vi "Main.vi"(11 "Error in":errorcluster) -> (15 "Error out":errorcluster)   [LabVIEW 2020, in "Simple calculator.lvlib"]
doc: "This System is an advanced calculator which is used to store and retrive data which we have already made."
uses:
  Simple calculator.lvlib
  Typedefs/Queue operations.ctl
  Typedefs/Data cluster.ctl
  Arithmetic Operations/Add/Add.lvclass
  Arithmetic Operations/Subtract/Subtract.lvclass
  Arithmetic Operations/Multiply/Multiply.lvclass
  Arithmetic Operations/Divide/Divide.lvclass
  Typedefs/User event operations.ctl
panel:
  in  "Delete":bool
  in  "Load":bool
  in  "Save":bool
  in  "Arithmetic operation":string(combo)
  in  "Add":bool
  in  "Operations added":string(tree)
  # "ADVANCED CALCULATOR"
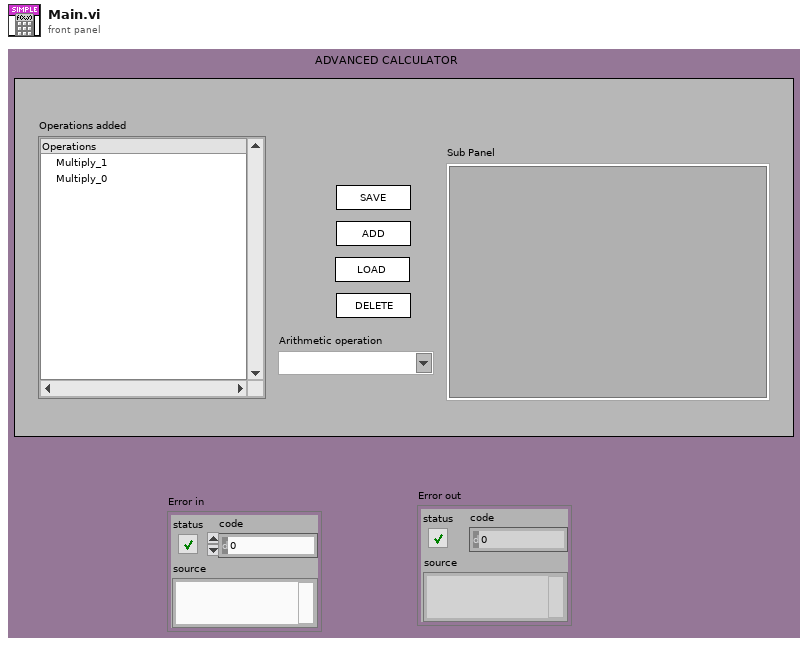
[diagram p1: front panel]
types:
  T1 = typedef "Simple calculator.lvlib/User event operations.ctl" = enum16{"Create", "Get Ref", "Generate ", "Destroy"}
  T2 = typedef "Simple calculator.lvlib/Data cluster.ctl" = cluster{"Load":bool, "Save":bool, "Add":bool, "Arithmetic operation":string, "Add Count":dbl, "Subtract Count":dbl, "Multiply Count":dbl, "Divide Count":dbl, "Delete Tag":string, "Add Object":refnum<class "Add.lvclass">[], "Sub Object":refnum<class "Subtract.lvclass">[], "Multiply Object":refnum<class "Multiply.lvclass">[], "Divide Object":refnum<class "Divide.lvclass">[], "Previous tag":i32, "Strict VI Ref":refnum<vi>, "Active Tag":i32, "Sub VI Refnum":refnum<vi>, "Multip VI Refnum":refnum<vi>, "Divide vi refnum":refnum<vi>}
  T3 = typedef "Simple calculator.lvlib/Queue operations.ctl" = enum16{"Create", "Enqueue", "Enstack", "Dequeue", "Flush", "Release"}
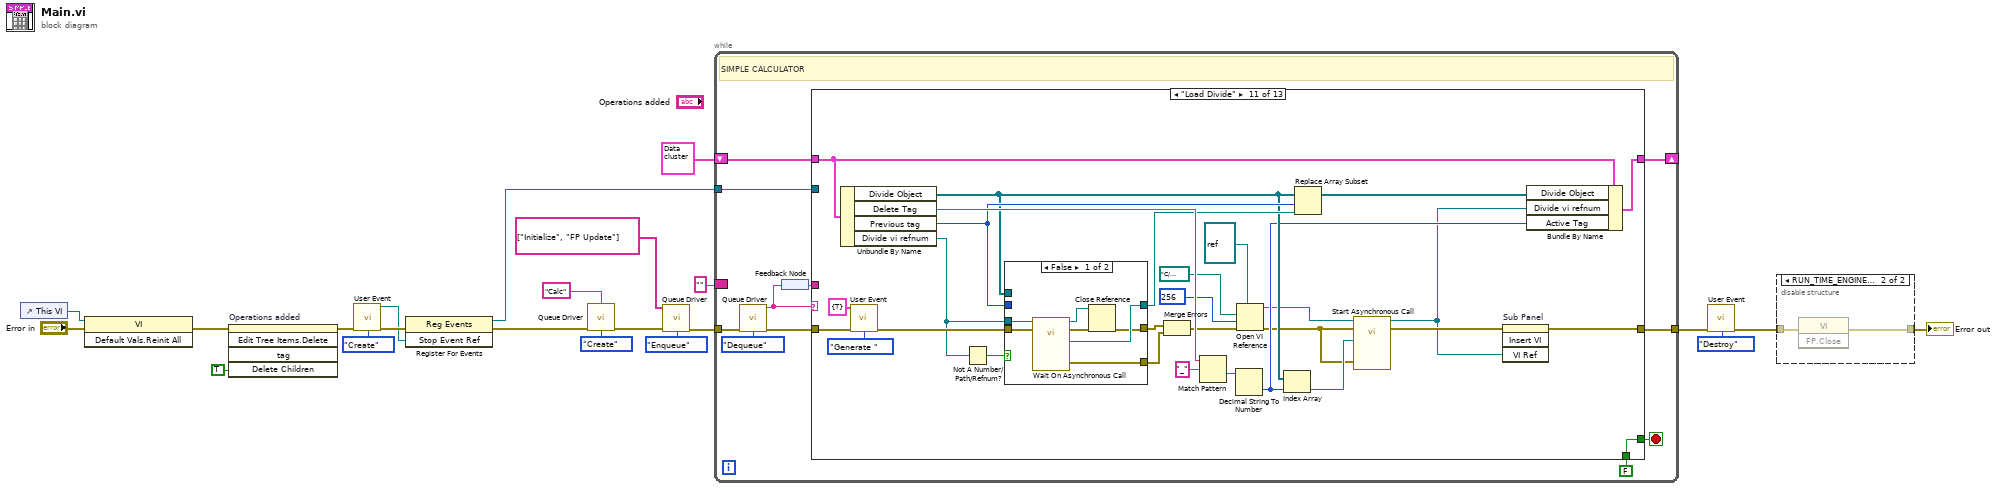
[diagram p0: block diagram]
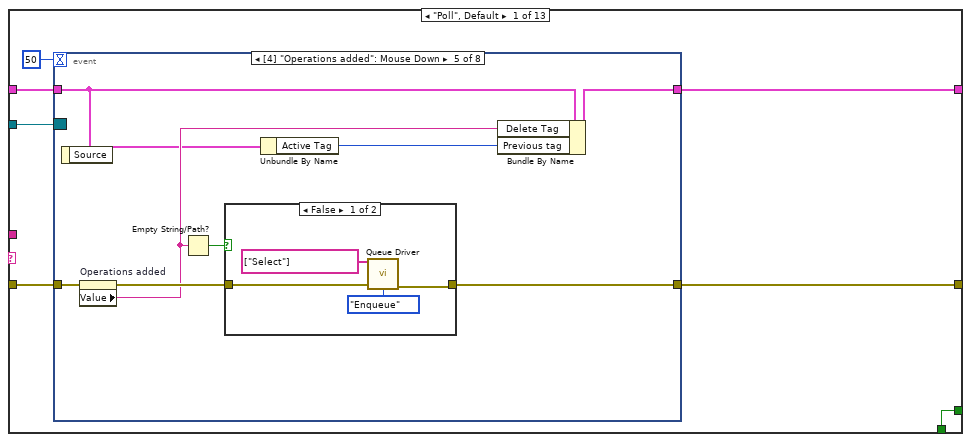
[diagram p3: hidden frame]
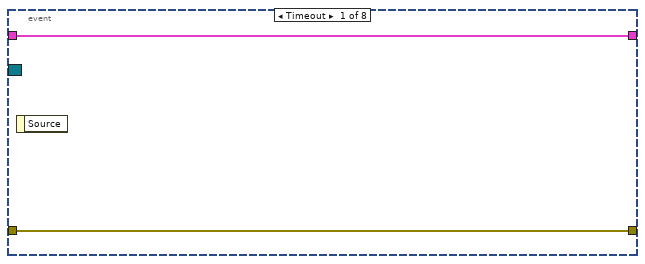
[diagram p4: hidden frame]
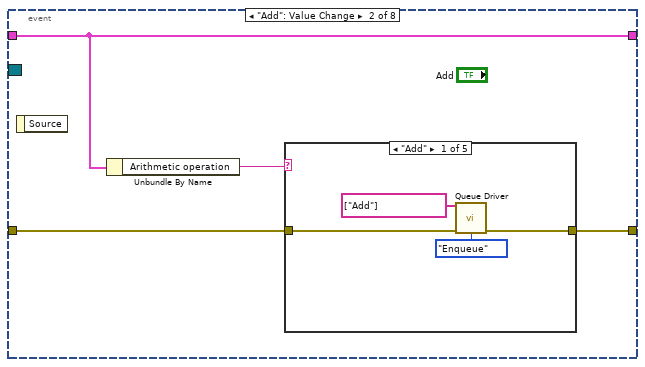
[diagram p5: hidden frame]
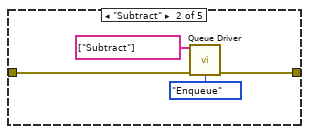
[diagram p6: hidden frame]
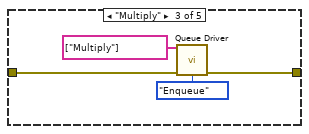
[diagram p7: hidden frame]
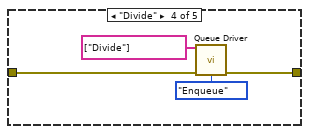
[diagram p8: hidden frame]
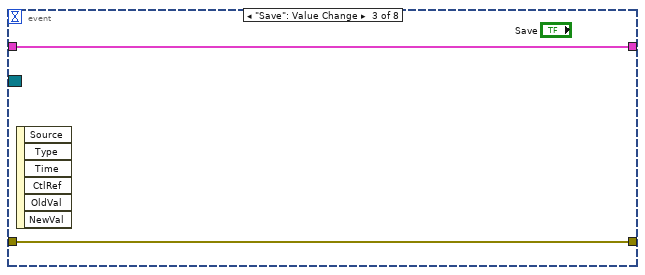
[diagram p10: hidden frame]
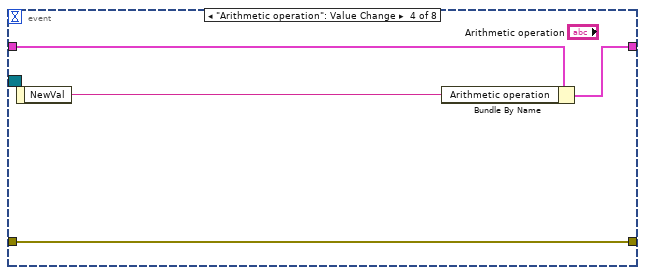
[diagram p11: hidden frame]
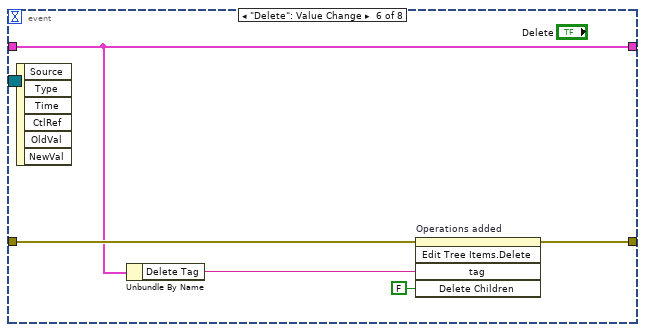
[diagram p13: hidden frame]
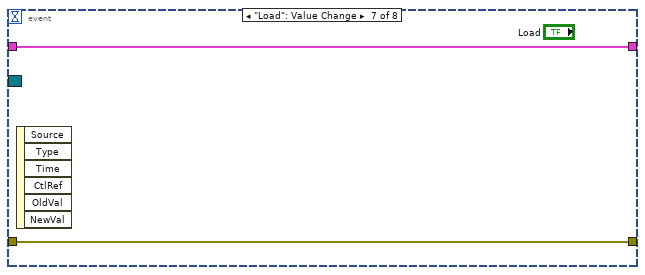
[diagram p14: hidden frame]
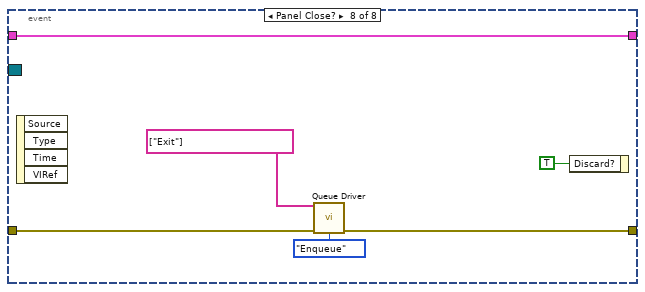
[diagram p15: hidden frame]
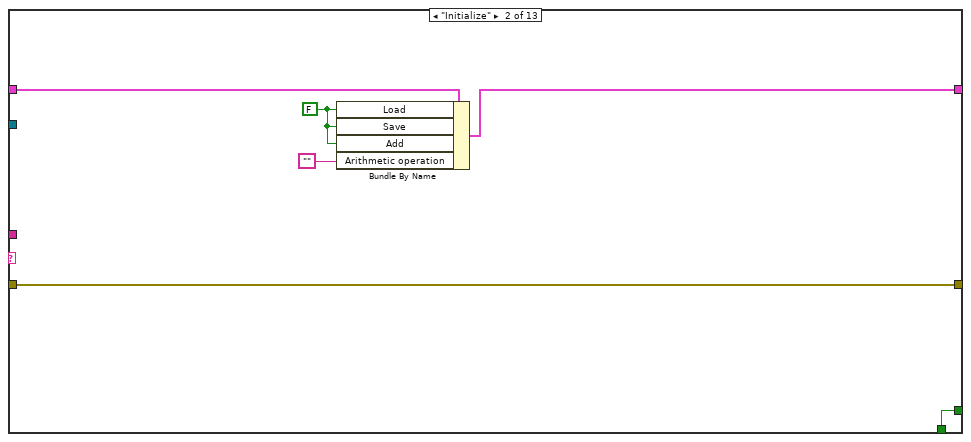
[diagram p16: hidden frame]
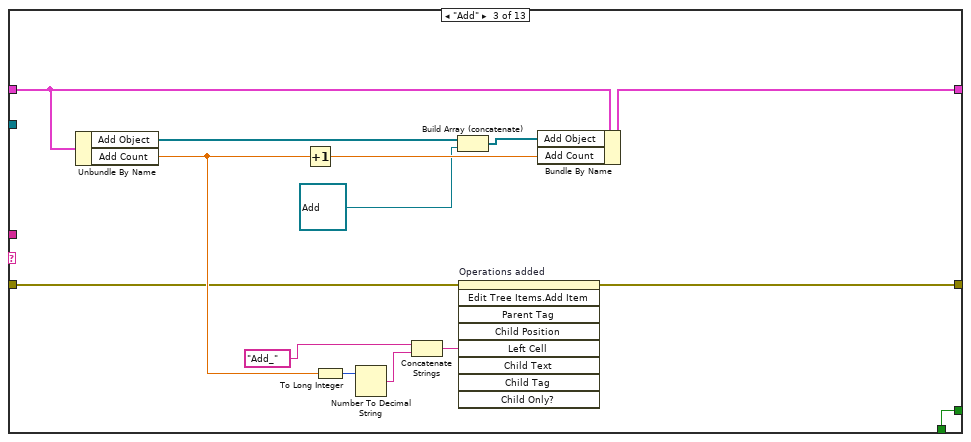
[diagram p17: hidden frame]
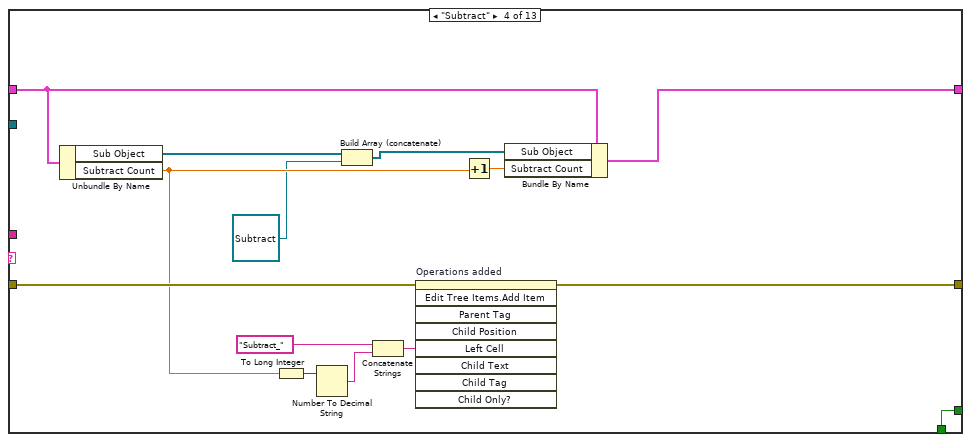
[diagram p18: hidden frame]
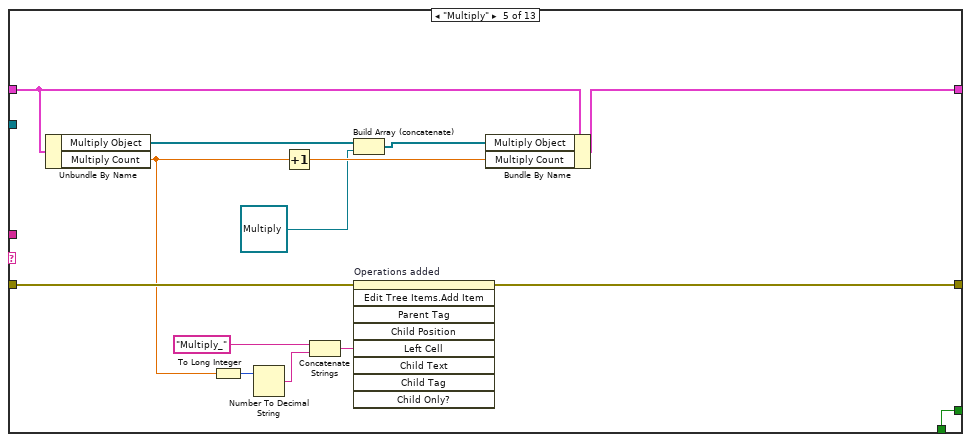
[diagram p19: hidden frame]
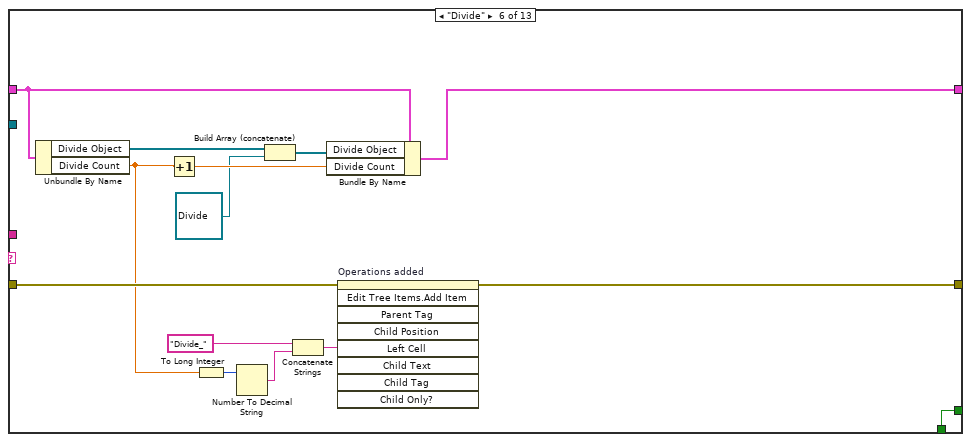
[diagram p20: hidden frame]
diagram:
  n1 = control-ref of="This VI"() -> (w21:refnum<vi>)
  n2 = invoke class="VI" method="Default Vals.Reinit All"(reference=w21, error in="Error in") -> (error out=w2:errorcluster)  [unwired: 1 in, 2 out]
  n3 = invoke on="Operations added" class="Tree (strict)" method="Edit Tree Items.Delete"(error in=w2, "Delete Children"=TRUE ("Delete Children?")) -> (error out=w1:errorcluster)  [unwired: 3 in, 4 out]
  n4 = call "User Event.vi"("Error in"=w1, "Operation"=User_event_operations."Create") -> ("Stop Event Ref"=w8:refnum<user-event>, "Error out"=w10:errorcluster)  [unwired: 12 in]
  n5 = register-events(error in=w10, w8) -> (reference out=w7:refnum<event-registration>, error out=w9:errorcluster)  [unwired: 1 in]
  n6 = call "Queue Driver.vi"("Name"="Calc", "Error in"=w9, "Operations"=Queue_operations."Create") -> ("Error out"=w17:errorcluster)  [unwired: 11 in, 1 out]
  n7 = call "Queue Driver.vi"("Enqueue states"=string[] ["Initialize", "FP Update"], "Error in"=w17, "Operations"=Queue_operations."Enqueue") -> ("Error out"=w15:errorcluster)  [unwired: 11 in, 1 out]
  n8 = while {
    tunnel: w15 -> [w32]
    border: "" ("Dequeued element") -> [_]
    tunnel: [w28] -> w5
    shift-right: [w25] -> _
    shift-left: T2 {"Load"=FALSE, "Save"=FALSE, "Add"=FALSE, "Arithmetic operation"="", "Add Count"=0.0, "Subtract Count"=0.0, "Multiply Count"=0.0, "Divide Count"=0.0, "Delete Tag"="", "Add Object"=[], "Sub Object"=[], "Multiply Object"=[], "Divide Object"=[], "Previous tag"=0, "Strict VI Ref"=refnum, "Active Tag"=0, "Sub VI Refnum"=refnum, "Multip VI Refnum"=refnum, "Divide vi refnum"=refnum} -> [w24]
    tunnel: w7 -> [w23]
    stop <- w27 stop-if-true
    # "SIMPLE CALCULATOR"
    n9 = call "Queue Driver.vi"("Error in"=w32, "Operations"=Queue_operations."Dequeue") -> ("Dequeued element"=w31:string, "Error out"=w29:errorcluster)  [unwired: 12 in]
    n10 = feedback-in #1(w31) -> ()
    n11 = feedback #1() -> (w30:string)
    n12 = case shown="\"Load Divide\"" w31 {
      tunnel: w30 -> [_ _ _ _ _ _ _ _ _ _ _ w346 _]
      tunnel: w29 -> [w40 w101 w103 w125 w142 w156 w159 w191 w223 w287 w327 w347 w363]
      tunnel: [w39 w101 w111 w124 w141 w155 w158 w187 w249 w262 w303 w343 w367] -> w28
      tunnel: [w38 w100 w115 w129 w143 w157 w164 w210 w250 w290 w330 w355 TRUE] -> w27
      tunnel: FALSE -> [w38 w100 w115 w129 w143 w157 w164 w210 w250 w290 w330 w355 _]
      tunnel: [w35 w98 w108 w119 w135 w149 w163 w201 w240 w274 w314 w342 w365] -> w25
      tunnel: w24 -> [w36 w99 w110 w120 w136 w150 w163 w202 w241 w275 w315 w342 w365]
      tunnel: w23 -> [w34 _ _ _ _ _ _ _ _ _ _ _ _]
      frame "Poll", Default {
        n13 = event shown="[4] \"Operations added\": Mouse Down" {
          selector: w34 -> [_ _ _ _ _ _ _ _]
          dyn-events: _ -> [_ _ _ _ _ _ _ _]
          timeout: 50 -> [_ _ _ _ _ _ _ _]
          tunnel: w40 -> [w42 w44 w65 w69 w77 w87 w89 w93]
          tunnel: [w42 w43 w65 w69 w70 w86 w89 w92] -> w39
          tunnel: w36 -> [w41 w46 w64 w68 w72 w84 w88 w90]
          tunnel: [w41 w46 w64 w66 w76 w84 w88 w90] -> w35
          event Timeout {
            n14 = event-data() -> ()  [unwired: 1 in, 1 out]
          }
          event "Add": Value Change {
            n15 = event-data() -> ()  [unwired: 1 in, 1 out]
            n16 = Unbundle By Name(w46) -> ("Arithmetic operation"=w45:string)
            n17 = case shown="\"Add\"" w45 {
              tunnel: w44 -> [w49 w52 w56 w60 w63]
              tunnel: [w47 w51 w55 w59 w63] -> w43
              frame "Add" {
                n18 = call "Queue Driver.vi"("Enqueue states"=string[] ["Add"], "Error in"=w49, "Operations"=Queue_operations."Enqueue") -> ("Error out"=w47:errorcluster)  [unwired: 11 in, 1 out]
              }
              frame "Subtract" {
                n19 = call "Queue Driver.vi"("Enqueue states"=string[] ["Subtract"], "Error in"=w52, "Operations"=Queue_operations."Enqueue") -> ("Error out"=w51:errorcluster)  [unwired: 11 in, 1 out]
              }
              frame "Multiply" {
                n20 = call "Queue Driver.vi"("Enqueue states"=string[] ["Multiply"], "Error in"=w56, "Operations"=Queue_operations."Enqueue") -> ("Error out"=w55:errorcluster)  [unwired: 11 in, 1 out]
              }
              frame "Divide" {
                n21 = call "Queue Driver.vi"("Enqueue states"=string[] ["Divide"], "Error in"=w60, "Operations"=Queue_operations."Enqueue") -> ("Error out"=w59:errorcluster)  [unwired: 11 in, 1 out]
              }
              frame "", Default {
              }
            }
          }
          event "Save": Value Change {
            n22 = event-data() -> ()  [unwired: 1 in, 6 out]
          }
          event "Arithmetic operation": Value Change {
            n23 = event-data() -> ("NewVal"=w67:string)  [unwired: 1 in]
            n24 = Bundle By Name(cluster=w68, "Arithmetic operation"=w67) -> (w66:T2)
          }
          event "Operations added": Mouse Down {
            n25 = event-data() -> ()  [unwired: 1 in, 1 out]
            n26 = property on="Operations added" class="Tree (strict)"(error in=w77) -> (error out=w74:errorcluster, "Value"=w73:string)  [unwired: 1 in, 1 out]
            n27 = Empty String/Path?(string/path=w73) -> (empty?=w75:bool)
            n28 = case shown="False" w75 {
              tunnel: [w79 w82] -> w70
              tunnel: w74 -> [w80 w82]
              frame False {
                n29 = call "Queue Driver.vi"("Enqueue states"=string[] ["Select"], "Error in"=w80, "Operations"=Queue_operations."Enqueue") -> ("Error out"=w79:errorcluster)  [unwired: 11 in, 1 out]
              }
              frame True {
              }
            }
            n30 = Unbundle By Name(w72) -> ("Active Tag"=w71:i32)
            n31 = Bundle By Name(cluster=w72, "Delete Tag"=w73, "Previous tag"=w71) -> (w76:T2)
          }
          event "Delete": Value Change {
            n32 = event-data() -> ()  [unwired: 1 in, 6 out]
            n33 = Unbundle By Name(w84) -> ("Delete Tag"=w83:string)
            n34 = invoke on="Operations added" class="Tree (strict)" method="Edit Tree Items.Delete"(error in=w87, "tag"=w83, "Delete Children"=FALSE ("Delete Children?")) -> (error out=w86:errorcluster)  [unwired: 2 in, 4 out]
          }
          event "Load": Value Change {
            n35 = event-data() -> ()  [unwired: 1 in, 6 out]
          }
          event Panel Close? {
            n36 = event-data() -> ()  [unwired: 1 in, 4 out]
            n37 = call "Queue Driver.vi"("Enqueue states"=string[] ["Exit"], "Error in"=w93, "Operations"=Queue_operations."Enqueue") -> ("Error out"=w92:errorcluster)  [unwired: 11 in, 1 out]
            n38 = event-data("Discard?"=TRUE) -> ()  [unwired: 1 in, 1 out]
          }
        }
      }
      frame "Initialize" {
        w97 = FALSE ("Load")
        n39 = Bundle By Name(cluster=w99, "Load"=w97, "Save"=w97, "Add"=w97, "Arithmetic operation"="") -> (w98:T2)
      }
      frame "Add" {
        n40 = Unbundle By Name(w110) -> ("Add Object"=w105:refnum<class "Add.lvclass">[], "Add Count"=w107:dbl)
        n41 = Increment(x=w107) -> (x+1=w109:dbl)
        n42 = To Long Integer(number=w107) -> (32bit integer=w114:i32)
        n43 = Number To Decimal String(number=w114) -> (decimal integer string=w113:string)  [unwired: 1 in]
        n44 = Concatenate Strings("Add_" ("Arithmetic operation"), w113) -> (w112:string)
        n45 = Build Array (concatenate)(w105, refnum<class "Add.lvclass"> refnum ("Add.lvclass")) -> (w104:refnum<class "Add.lvclass">[])
        n46 = invoke on="Operations added" class="Tree (strict)" method="Edit Tree Items.Add Item"(error in=w103, "Left Cell"=w112) -> (error out=w111:errorcluster)  [unwired: 7 in, 8 out]
        n47 = Bundle By Name(cluster=w110, "Add Object"=w104, "Add Count"=w109) -> (w108:T2)
      }
      frame "Subtract" {
        n48 = Unbundle By Name(w120) -> ("Sub Object"=w118:refnum<class "Subtract.lvclass">[], "Subtract Count"=w122:dbl)
        n49 = To Long Integer(number=w122) -> (32bit integer=w128:i32)
        n50 = Number To Decimal String(number=w128) -> (decimal integer string=w126:string)  [unwired: 1 in]
        n51 = Build Array (concatenate)(w118, refnum<class "Subtract.lvclass"> refnum ("Subtract.lvclass")) -> (w116:refnum<class "Subtract.lvclass">[])
        n52 = Concatenate Strings("Subtract_" ("string"), w126) -> (w123:string)
        n53 = invoke on="Operations added" class="Tree (strict)" method="Edit Tree Items.Add Item"(error in=w125, "Left Cell"=w123) -> (error out=w124:errorcluster)  [unwired: 7 in, 8 out]
        n54 = Increment(x=w122) -> (x+1=w121:dbl)
        n55 = Bundle By Name(cluster=w120, "Sub Object"=w116, "Subtract Count"=w121) -> (w119:T2)
      }
      frame "Multiply" {
        n56 = Unbundle By Name(w136) -> ("Multiply Object"=w132:refnum<class "Multiply.lvclass">[], "Multiply Count"=w133:dbl)
        n57 = To Long Integer(number=w133) -> (32bit integer=w140:i32)
        n58 = Number To Decimal String(number=w140) -> (decimal integer string=w138:string)  [unwired: 1 in]
        n59 = Increment(x=w133) -> (x+1=w134:dbl)
        n60 = Concatenate Strings("Multiply_" ("string"), w138) -> (w137:string)
        n61 = Build Array (concatenate)(w132, refnum<class "Multiply.lvclass"> refnum ("Multiply.lvclass")) -> (w130:refnum<class "Multiply.lvclass">[])
        n62 = invoke on="Operations added" class="Tree (strict)" method="Edit Tree Items.Add Item"(error in=w142, "Left Cell"=w137) -> (error out=w141:errorcluster)  [unwired: 7 in, 8 out]
        n63 = Bundle By Name(cluster=w136, "Multiply Object"=w130, "Multiply Count"=w134) -> (w135:T2)
      }
      frame "Divide" {
        n64 = Unbundle By Name(w150) -> ("Divide Object"=w146:refnum<class "Divide.lvclass">[], "Divide Count"=w147:dbl)
        n65 = Increment(x=w147) -> (x+1=w148:dbl)
        n66 = To Long Integer(number=w147) -> (32bit integer=w154:i32)
        n67 = Number To Decimal String(number=w154) -> (decimal integer string=w152:string)  [unwired: 1 in]
        n68 = Build Array (concatenate)(w146, refnum<class "Divide.lvclass"> refnum ("Divide.lvclass")) -> (w144:refnum<class "Divide.lvclass">[])
        n69 = Concatenate Strings("Divide_" ("string"), w152) -> (w151:string)
        n70 = Bundle By Name(cluster=w150, "Divide Object"=w144, "Divide Count"=w148) -> (w149:T2)
        n71 = invoke on="Operations added" class="Tree (strict)" method="Edit Tree Items.Add Item"(error in=w156, "Left Cell"=w151) -> (error out=w155:errorcluster)  [unwired: 7 in, 8 out]
      }
      frame "Select" {
        n72 = Unbundle By Name(w163) -> ("Delete Tag"=w161:string)
        n73 = Match Pattern(string=w161, regular expression="_") -> (before substring=w160:string)  [unwired: 1 in, 3 out]
        n74 = case shown="\"Divide\"" w160 {
          tunnel: w159 -> [w167 w170 w173 w178 w181]
          tunnel: [w166 w169 w174 w177 w181] -> w158
          frame "Add" {
            n75 = call "Queue Driver.vi"("Enqueue states"=string[] ["Load Add"], "Error in"=w167, "Operations"=Queue_operations."Enqueue") -> ("Error out"=w166:errorcluster)  [unwired: 11 in, 1 out]
          }
          frame "Subtract" {
            n76 = call "Queue Driver.vi"("Enqueue states"=string[] ["Load Sub"], "Error in"=w170, "Operations"=Queue_operations."Enqueue") -> ("Error out"=w169:errorcluster)  [unwired: 11 in, 1 out]
          }
          frame "Multiply" {
            n77 = call "Queue Driver.vi"("Enqueue states"=string[] ["Load Multiply"], "Error in"=w173, "Operations"=Queue_operations."Enqueue") -> ("Error out"=w174:errorcluster)  [unwired: 11 in, 1 out]
          }
          frame "Divide" {
            n78 = call "Queue Driver.vi"("Enqueue states"=string[] ["Load Divide"], "Error in"=w178, "Operations"=Queue_operations."Enqueue") -> ("Error out"=w177:errorcluster)  [unwired: 11 in, 1 out]
          }
          frame "", Default {
          }
        }
      }
      frame "Load Add" {
        n79 = Unbundle By Name(w202) -> ("Add Object"=w189:refnum<class "Add.lvclass">[], "Delete Tag"=w203:string, "Previous tag"=w188:i32, "Strict VI Ref"=w194:refnum<vi>)
        n80 = call "User Event.vi"("Stop Event"=cluster{"Stop":bool} {"Stop"=TRUE}, "Error in"=w191, "Operation"=User_event_operations."Generate ") -> ("Error out"=w190:errorcluster)  [unwired: 11 in, 1 out]
        n81 = Not A Number/Path/Refnum?(number/path/refnum=w194) -> (NaN/Path/Refnum?=w196:bool)
        n82 = case shown="True" w196 {
          tunnel: w190 -> [w217 w221]
          tunnel: [w216 w221] -> w198
          tunnel: [w214 w221] -> w197
          tunnel: [w212 w218] -> w195
          tunnel: w188 -> [_ w220]
          tunnel: w189 -> [_ w219]
          tunnel: w194 -> [w211 _]
          frame False {
            n83 = call-by-ref "Wait On Asynchronous Call"(reference=w211, error in=w217) -> (reference out=w213:refnum<vi>, error out=w215:errorcluster, 0:"error out"=w216:errorcluster, "Add out"=w212:refnum<class "Add.lvclass">)  [unwired: 10 in]
            n84 = Close Reference(reference=w213, error in (no error)=w215) -> (error out=w214:errorcluster)
          }
          frame True {
            n85 = Index Array(array=w219, index=w220) -> (element=w218:refnum<class "Add.lvclass">)
          }
        }
        n86 = Merge Errors(w197, w198) -> (w199:errorcluster)
        n87 = Match Pattern(string=w203, regular expression="_") -> (after substring=w204:string)  [unwired: 1 in, 3 out]
        n88 = Decimal String To Number(string=w204) -> (number=w186:i32)  [unwired: 2 in, 1 out]
        n89 = Index Array(array=w189, index=w186) -> (element=w182:refnum<class "Add.lvclass">)
        n90 = Open VI Reference(type specifier VI Refnum (for type only)=refnum<vi> refnum, vi path=path "C:/Users/khishore.kumar/Khishore/labview_tips_2024/src/Assignment 25/Arithmetic Operations/Add/Method/UI.vi", options=256, error in (no error)=w199) -> (vi reference=w184:refnum<vi>, error out=w208:errorcluster)  [unwired: 2 in]
        n91 = Replace Array Subset(array=w189, new element=w195, index=w188) -> (w200:refnum<class "Add.lvclass">[])
        n92 = call-by-ref "Start Asynchronous Call"(reference=w184, error in=w208, "Add in"=w182) -> (reference out=w185:refnum<vi>, error out=w207:errorcluster)  [unwired: 9 in, 2 out]
        n93 = invoke on="Sub Panel" class="SubPnl" method="Insert VI"(error in=w207, "VI Ref"=w185) -> (error out=w187:errorcluster)  [unwired: 2 in, 3 out]
        n94 = Bundle By Name(cluster=w202, "Add Object"=w200, "Strict VI Ref"=w185, "Active Tag"=w186) -> (w201:T2)
      }
      frame "Load Sub" {
        n95 = Unbundle By Name(w241) -> ("Sub Object"=w238:refnum<class "Subtract.lvclass">[], "Delete Tag"=w242:string, "Previous tag"=w239:i32, "Sub VI Refnum"=w247:refnum<vi>)
        n96 = call "User Event.vi"("Stop Event"=cluster{"Stop":bool} {"Stop"=TRUE}, "Error in"=w223, "Operation"=User_event_operations."Generate ") -> ("Error out"=w222:errorcluster)  [unwired: 11 in, 1 out]
        n97 = Not A Number/Path/Refnum?(number/path/refnum=w247) -> (NaN/Path/Refnum?=w248:bool)
        n98 = case shown="True" w248 {
          tunnel: w222 -> [w256 w258]
          tunnel: [w257 w258] -> w246
          tunnel: w238 -> [_ w261]
          tunnel: w239 -> [_ w260]
          tunnel: [w252 w259] -> w237
          tunnel: w247 -> [w253 _]
          tunnel: [w251 w258] -> w245
          frame False {
            n99 = call-by-ref "Wait On Asynchronous Call"(reference=w253, error in=w256) -> (reference out=w254:refnum<vi>, error out=w255:errorcluster, 0:"error out"=w251:errorcluster, "Subtract out"=w252:refnum<class "Subtract.lvclass">)  [unwired: 10 in]
            n100 = Close Reference(reference=w254, error in (no error)=w255) -> (error out=w257:errorcluster)
          }
          frame True {
            n101 = Index Array(array=w261, index=w260) -> (element=w259:refnum<class "Subtract.lvclass">)
          }
        }
        n102 = Merge Errors(w246, w245) -> (w235:errorcluster)
        n103 = Match Pattern(string=w242, regular expression="_") -> (after substring=w243:string)  [unwired: 1 in, 3 out]
        n104 = Decimal String To Number(string=w243) -> (number=w226:i32)  [unwired: 2 in, 1 out]
        n105 = Index Array(array=w238, index=w226) -> (element=w230:refnum<class "Subtract.lvclass">)
        n106 = Open VI Reference(type specifier VI Refnum (for type only)=refnum<vi> refnum, vi path=path "C:/Users/khishore.kumar/Khishore/labview_tips_2024/src/Assignment 25/Arithmetic Operations/Subtract/Method/UI.vi", options=256, error in (no error)=w235) -> (vi reference=w231:refnum<vi>, error out=w229:errorcluster)  [unwired: 2 in]
        n107 = Replace Array Subset(array=w238, new element=w237, index=w239) -> (w236:refnum<class "Subtract.lvclass">[])
        n108 = call-by-ref "Start Asynchronous Call"(reference=w231, error in=w229, 8:"error in (no error)"=w229, "Subtract in"=w230) -> (reference out=w227:refnum<vi>, error out=w228:errorcluster)  [unwired: 8 in, 2 out]
        n109 = Bundle By Name(cluster=w241, "Sub Object"=w236, "Sub VI Refnum"=w227, "Active Tag"=w226) -> (w240:T2)
        n110 = invoke on="Sub Panel" class="SubPnl" method="Insert VI"(error in=w228, "VI Ref"=w227) -> (error out=w249:errorcluster)  [unwired: 2 in, 3 out]
      }
      frame "Load Multiply" {
        n111 = call "User Event.vi"("Stop Event"=cluster{"Stop":bool} {"Stop"=TRUE}, "Error in"=w287, "Operation"=User_event_operations."Generate ") -> ("Error out"=w285:errorcluster)  [unwired: 11 in, 1 out]
        n112 = Unbundle By Name(w275) -> ("Multiply Object"=w281:refnum<class "Multiply.lvclass">[], "Delete Tag"=w276:string, "Previous tag"=w279:i32, "Multip VI Refnum"=w284:refnum<vi>)
        n113 = Not A Number/Path/Refnum?(number/path/refnum=w284) -> (NaN/Path/Refnum?=w286:bool)
        n114 = case shown="True" w286 {
          tunnel: w281 -> [_ w301]
          tunnel: w279 -> [_ w300]
          tunnel: w285 -> [w297 w299]
          tunnel: w284 -> [w296 _]
          tunnel: [w293 w299] -> w282
          tunnel: [w292 w299] -> w283
          tunnel: [w291 w298] -> w280
          frame False {
            n115 = call-by-ref "Wait On Asynchronous Call"(reference=w296, error in=w297) -> (reference out=w295:refnum<vi>, error out=w294:errorcluster, 0:"error out"=w293:errorcluster, "Multiply out"=w291:refnum<class "Multiply.lvclass">)  [unwired: 10 in]
            n116 = Close Reference(reference=w295, error in (no error)=w294) -> (error out=w292:errorcluster)
          }
          frame True {
            n117 = Index Array(array=w301, index=w300) -> (element=w298:refnum<class "Multiply.lvclass">)
          }
        }
        n118 = Merge Errors(w283, w282) -> (w270:errorcluster)
        n119 = Replace Array Subset(array=w281, new element=w280, index=w279) -> (w272:refnum<class "Multiply.lvclass">[])
        n120 = Match Pattern(string=w276, regular expression="_") -> (after substring=w277:string)  [unwired: 1 in, 3 out]
        n121 = Open VI Reference(type specifier VI Refnum (for type only)=refnum<vi> refnum, vi path=path "C:/Users/khishore.kumar/Khishore/labview_tips_2024/src/Assignment 25/Arithmetic Operations/Multiply/Method/UI.vi", options=256, error in (no error)=w270) -> (vi reference=w267:refnum<vi>, error out=w265:errorcluster)  [unwired: 2 in]
        n122 = Decimal String To Number(string=w277) -> (number=w273:i32)  [unwired: 2 in, 1 out]
        n123 = Index Array(array=w272, index=w273) -> (element=w266:refnum<class "Multiply.lvclass">)
        n124 = call-by-ref "Start Asynchronous Call"(reference=w267, error in=w265, 8:"error in (no error)"=w265, "Multiply in"=w266) -> (reference out=w263:refnum<vi>, error out=w264:errorcluster)  [unwired: 8 in, 2 out]
        n125 = invoke on="Sub Panel" class="SubPnl" method="Insert VI"(error in=w264, "VI Ref"=w263) -> (error out=w262:errorcluster)  [unwired: 2 in, 3 out]
        n126 = Bundle By Name(cluster=w275, "Multiply Object"=w272, "Multip VI Refnum"=w263, "Active Tag"=w273) -> (w274:T2)
      }
      frame "Load Divide" {
        n127 = Unbundle By Name(w315) -> ("Divide Object"=w316:refnum<class "Divide.lvclass">[], "Delete Tag"=w319:string, "Previous tag"=w318:i32, "Divide vi refnum"=w324:refnum<vi>)
        n128 = call "User Event.vi"("Stop Event"=cluster{"Stop":bool} {"Stop"=TRUE}, "Error in"=w327, "Operation"=User_event_operations."Generate ") -> ("Error out"=w325:errorcluster)  [unwired: 11 in, 1 out]
        n129 = Not A Number/Path/Refnum?(number/path/refnum=w324) -> (NaN/Path/Refnum?=w326:bool)
        n130 = case shown="False" w326 {
          tunnel: w316 -> [_ w341]
          tunnel: w318 -> [_ w340]
          tunnel: w325 -> [w337 w339]
          tunnel: w324 -> [w336 _]
          tunnel: [w333 w338] -> w317
          tunnel: [w332 w339] -> w323
          tunnel: [w331 w339] -> w322
          frame False {
            n131 = call-by-ref "Wait On Asynchronous Call"(reference=w336, error in=w337) -> (reference out=w334:refnum<vi>, error out=w335:errorcluster, 0:"error out"=w331:errorcluster, "Divide out"=w333:refnum<class "Divide.lvclass">)  [unwired: 10 in]
            n132 = Close Reference(reference=w334, error in (no error)=w335) -> (error out=w332:errorcluster)
          }
          frame True {
            n133 = Index Array(array=w341, index=w340) -> (element=w338:refnum<class "Divide.lvclass">)
          }
        }
        n134 = Merge Errors(w323, w322) -> (w311:errorcluster)
        n135 = Match Pattern(string=w319, regular expression="_") -> (after substring=w321:string)  [unwired: 1 in, 3 out]
        n136 = Decimal String To Number(string=w321) -> (number=w312:i32)  [unwired: 2 in, 1 out]
        n137 = Open VI Reference(type specifier VI Refnum (for type only)=refnum<vi> refnum, vi path=path "C:/Users/khishore.kumar/Khishore/labview_tips_2024/src/Assignment 25/Arithmetic Operations/Divide/Method/UI.vi", options=256, error in (no error)=w311) -> (vi reference=w307:refnum<vi>, error out=w305:errorcluster)  [unwired: 2 in]
        n138 = Index Array(array=w316, index=w312) -> (element=w306:refnum<class "Divide.lvclass">)
        n139 = Replace Array Subset(array=w316, new element=w317, index=w318) -> (w313:refnum<class "Divide.lvclass">[])
        n140 = call-by-ref "Start Asynchronous Call"(reference=w307, error in=w305, "Error in"=w305, "Divide in"=w306) -> (reference out=w302:refnum<vi>, error out=w304:errorcluster)  [unwired: 8 in, 2 out]
        n141 = invoke on="Sub Panel" class="SubPnl" method="Insert VI"(error in=w304, "VI Ref"=w302) -> (error out=w303:errorcluster)  [unwired: 2 in, 3 out]
        n142 = Bundle By Name(cluster=w315, "Divide Object"=w313, "Divide vi refnum"=w302, "Active Tag"=w312) -> (w314:T2)
      }
      frame "Error" {
        # "Handle the error occurred"
        n143 = Unbundle By Name(w347) -> ("code"=w352:i32, "source"=w351:string)
        n144 = call <vilib>:"Clear Errors.vi"("error in (no error)"=w347, "specific error code to clear (0: all)"=w352) -> ("error out"=w354:errorcluster)  [unwired: 4 in, 1 out]
        n145 = Format Into String(format string="Error occurred in state \"%s\"!!\nError Code: %d\nError Source: %s\n\nDo you wish to continue?", error in=w354, w346, w352, w351) -> (resulting string=w350:string, error out=w344:errorcluster)  [unwired: 1 in]
        n146 = Two Button Dialog(message=w350, 1:"Exit" ("F button name (\"Cancel\")"), 2:"Continue" ("T button name (\"OK\")")) -> (T button?=w345:bool)
        n147 = case shown="False" w345 {
          tunnel: w344 -> [w358 w360]
          tunnel: [w357 w360] -> w343
          frame False {
            # "Exit"
            n148 = call "Queue Driver.vi"("Enqueue states"=string[] ["Exit"], "Error in"=w358, "Operations"=Queue_operations."Enqueue") -> ("Error out"=w357:errorcluster)  [unwired: 11 in, 1 out]
          }
          frame True {
            # "Continue"
          }
        }
      }
      frame "Exit" {
        # "Flush ,Release and terminate the machine."
        n149 = call "User Event.vi"("Stop Event"=cluster{"Stop":bool} {"Stop"=TRUE}, "Error in"=w363, "Operation"=User_event_operations."Generate ") -> ("Error out"=w362:errorcluster)  [unwired: 11 in, 1 out]
        n150 = call "Queue Driver.vi"("Error in"=w362, "Operations"=Queue_operations."Flush") -> ("Error out"=w368:errorcluster)  [unwired: 12 in, 1 out]
        n151 = call "Queue Driver.vi"("Error in"=w368, "Operations"=Queue_operations."Release") -> ("Error out"=w367:errorcluster)  [unwired: 12 in, 1 out]
      }
    }
  }
  n152 = call "User Event.vi"("Error in"=w5, "Operation"=User_event_operations."Destroy") -> ("Error out"=w4:errorcluster)  [unwired: 12 in, 1 out]
  n153 = disable-structure shown="RUN_TIME_ENGINE==True" {
    disable-tunnel: w4 -> [w371 w373]
    disable-tunnel: [w371 w372] -> w13
    frame condition #0 (active) {
    }
    frame condition #1 {
      n154 = invoke class="VI" method="FP.Close"(error in=w373) -> (error out=w372:errorcluster)  [unwired: 2 in, 2 out]
    }
  }
  "Error out" <- w13
